vi "Add Calibration.vi"(5 "Temperature Sensors":cluster{"name":string, "reading":dbl}[](array[cluster]), 7 "Calibration Date":timestamp format="%<%x>T", 8 "error in":errorcluster, 10 "Serial Number":string, 11 "NI Skyline Configuration HTTP in":refnum<class "NI Skyline Configuration HTTP.lvclass">) -> (0 "error out":errorcluster, 3 "NI Skyline Configuration HTTP out":refnum<class "NI Skyline Configuration HTTP.lvclass">)   [LabVIEW 2020]
uses:
  <vilib>/Skyline/Configuration/Configuration HTTP_class/NI Skyline Configuration HTTP.lvclass
  <vilib>/Skyline/Configuration/Configuration HTTP_class/NI Skyline Configuration HTTP.lvclass/NI Skyline Configuration HTTP.ctl
  <vilib>/Skyline/Configuration/Configuration HTTP_class/Read Server URL.vi
  <vilib>/httpClient/POSTBuffer.vi
  <vilib>/httpClient/LabVIEWHTTPClient.lvlib
  <vilib>/addons/_JKI.lib/Serialization/JSON/JKI JSON Serialization.lvlib
panel:
  out "response headers":string
  out "response body":string
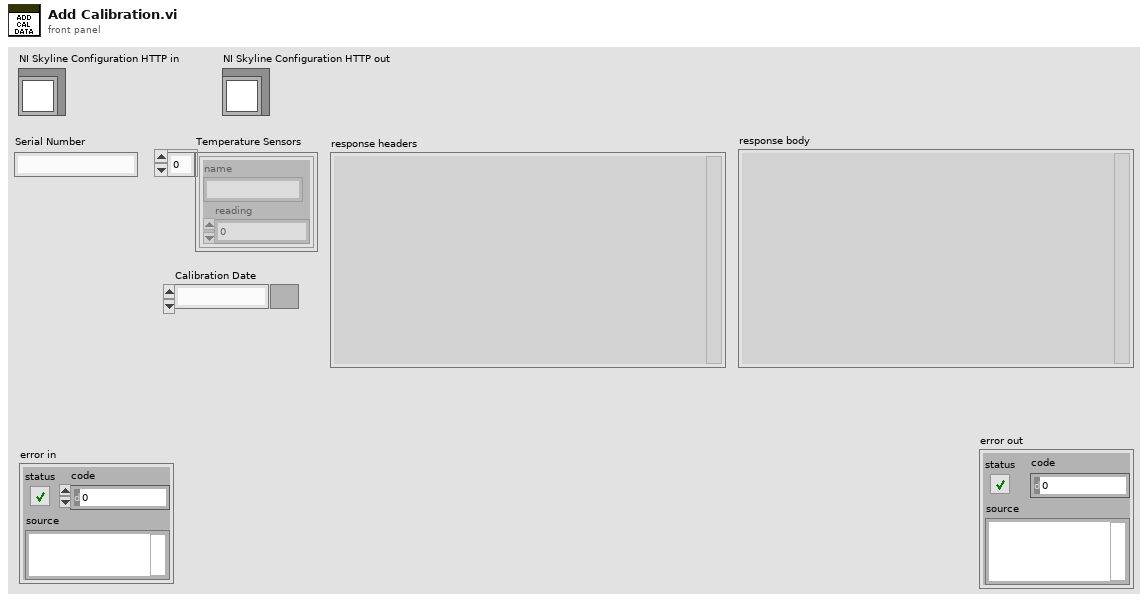
[diagram p1: front panel]
types:
  T1 = typedef "Assets.ctl" = cluster{"assets":T2[], "totalCount":u64}
  T2 = typedef "Asset.ctl" = cluster{"modelName":string, "modelNumber":u64, "serialNumber":string, "vendorName":string, "vendorNumber":u64, "busType":string, "name":string, "assetType":string, "discoveryType":string, "firmwareVersion":string, "hardwareVersion":string, "visaResourceName":string, "temperatureSensors":string[], "supportsSelfCalibration":bool, "supportsExternalCalibration":bool, "isNIAsset?":bool, "id":string, "location":cluster{"minionId":string, "parent":string, "resourceUri":string, "slotNumber":u64, "systemName":string, "state":cluster{"assetPresence":string, "systemConnection":string}}, "calibrationStatus":string, "isSystemController":bool, "externalCalibration":T3, "workspace":string, "keywords":string[], "lastUpdatedTimestamp":string}
  T3 = typedef "externalCalibration.ctl" = cluster{"temperatureSensors":cluster{"name":string, "reading":dbl}[], "isLimited":bool, "date":timestamp, "recommendedInterval":i32, "nextRecommendedDate":timestamp, "comments":string, "entrytype":string, "operator":cluster{"displayName":string, "userID":string}}
  T4 = typedef "LabVIEWHTTPClient.lvlib/ClientHandle.ctl" = refnum<k1>
  T5 = typedef "LVDateTimeRec.ctl" = cluster{"fractional second":dbl, "second":i32, "minute":i32, "hour":i32, "day of month":i32, "month":i32, "year":i32, "day of week":i32, "day of year":i32, "DST":i32}
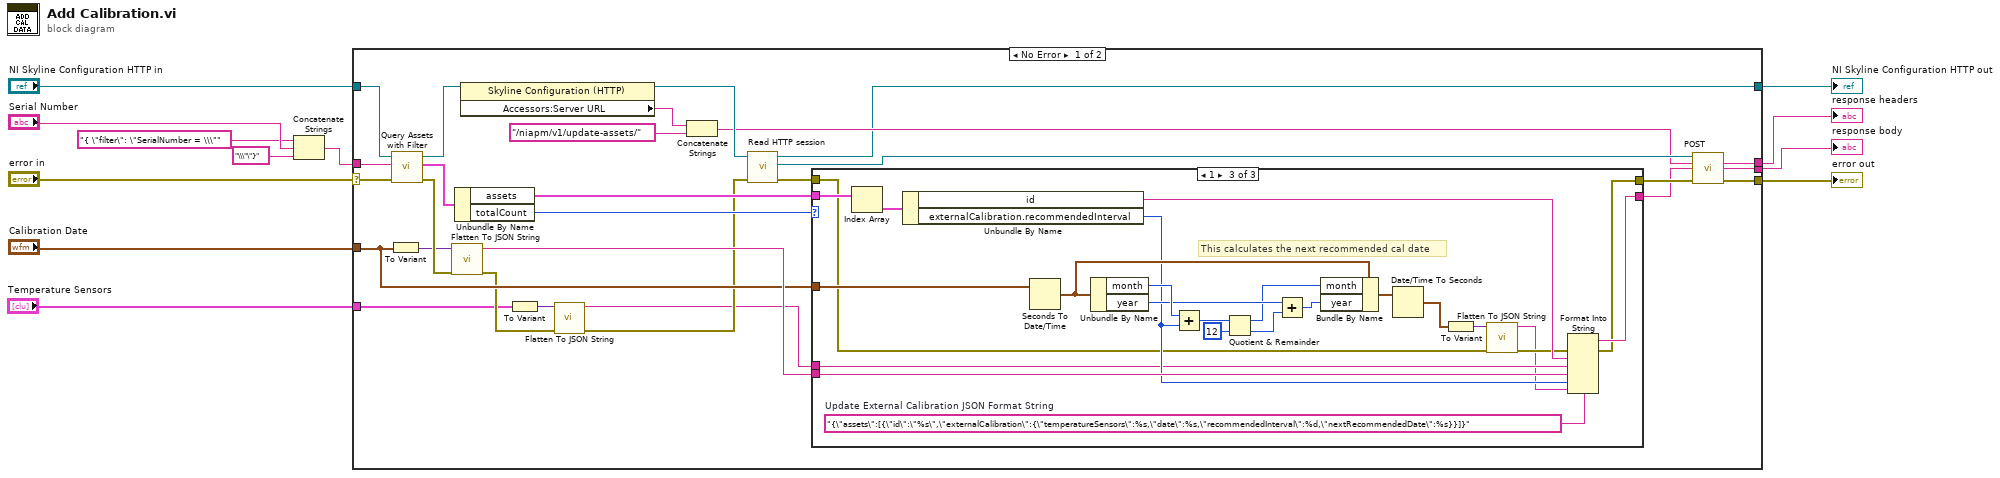
[diagram p0: block diagram]
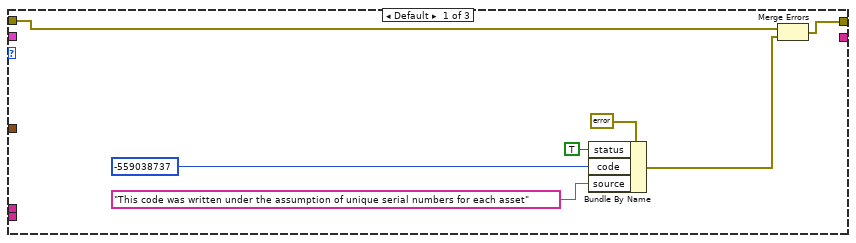
[diagram p2: hidden frame]
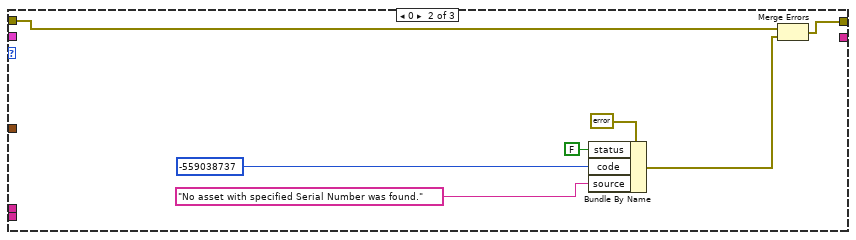
[diagram p3: hidden frame]
diagram:
  n1 = Concatenate Strings("{ \"filter\": \"SerialNumber = \\\"" ("string"), "Serial Number", "\\\"\"}" ("string")) -> (w8:string)
  n2 = case shown="No Error" "error in" {
    selector: "error in" -> [w27 w79]
    tunnel: "NI Skyline Configuration HTTP in" -> [w40 w80]
    tunnel: w8 -> [w39 _]
    tunnel: [w32 w79] -> w7
    tunnel: [w31 _] -> w6
    tunnel: [w30 w80] -> w5
    tunnel: "Calibration Date" -> [w18 _]
    tunnel: [w28 _] -> w4
    tunnel: "Temperature Sensors" -> [w14 _]
    frame No Error {
      n3 = To Variant(anything=w18) -> (Variant=w19:variant)
      n4 = call "Query Assets with Filter.vi"("Error in"=w27, "Filter string"=w39, "NI Skyline Configuration HTTP in"=w40) -> ("Error out"=w20:errorcluster, "Assets"=w29:T1, "NI Skyline Configuration HTTP out"=w38:refnum<class "NI Skyline Configuration HTTP.lvclass">)  [unwired: 6 in]
      n5 = call <vilib>:"Flatten To JSON String.vi"("error in (no error)"=w20, "Variant"=w19) -> ("error out"=w17:errorcluster, "JSON String"=w21:string)  [unwired: 8 in]
      n6 = Unbundle By Name(w29) -> ("assets"=w26:T2[], "totalCount"=w25:u64)
      n7 = property class="Skyline Configuration (HTTP)"(reference=w38) -> (reference out=w35:refnum<class "NI Skyline Configuration HTTP.lvclass">, "Accessors:Server URL"=w37:string)  [unwired: 1 in, 1 out]
      n8 = To Variant(anything=w14) -> (Variant=w15:variant)
      n9 = call <vilib>:"Flatten To JSON String.vi"("error in (no error)"=w17, "Variant"=w15) -> ("error out"=w16:errorcluster, "JSON String"=w13:string)  [unwired: 8 in]
      n10 = Concatenate Strings(w37, "/niapm/v1/update-assets/" ("initial string")) -> (w33:string)
      n11 = call <vilib>:"Read HTTP session.vi"("error in (no error)"=w16, "HTTP configuration in"=w35) -> ("error out"=w24:errorcluster, "http session"=w34:T4, "HTTP configuration out"=w30:refnum<class "NI Skyline Configuration HTTP.lvclass">)  [unwired: 7 in]
      n12 = case shown="1" w25 {
        tunnel: w26 -> [_ _ w78]
        tunnel: w18 -> [_ _ w66]
        tunnel: [_ _ w65] -> w22
        tunnel: w24 -> [w45 w52 w59]
        tunnel: [w44 w53 w64] -> w23
        tunnel: w21 -> [_ _ w63]
        tunnel: w13 -> [_ _ w61]
        frame Default {
          n13 = Bundle By Name(cluster=errorcluster {"status"=FALSE, "code"=0, "source"=""} ("error in (no error)"), "status"=TRUE, "code"=-559038737, "source"="This code was written under the assumption of unique serial numbers for each asset") -> (w47:errorcluster)
          n14 = Merge Errors(w45, w47) -> (w44:errorcluster)
        }
        frame 0 {
          n15 = Bundle By Name(cluster=errorcluster {"status"=FALSE, "code"=0, "source"=""} ("error in (no error)"), "status"=FALSE, "code"=-559038737, "source"="No asset with specified Serial Number was found.") -> (w51:errorcluster)
          n16 = Merge Errors(w52, w51) -> (w53:errorcluster)
        }
        frame 1 {
          w55 = "{\"assets\":[{\"id\":\"%s\",\"externalCalibration\":{\"temperatureSensors\":%s,\"date\":%s,\"recommendedInterval\":%d,\"nextRecommendedDate\":%s}}]}"  # Update External Calibration JSON Format String
          # "This calculates the next recommended cal date"
          n17 = Index Array(array=w78) -> (element=w77:T2)  [unwired: 1 in]
          n18 = Unbundle By Name(w77) -> ("id"=w67:string, "externalCalibration.recommendedInterval"=w62:i32)
          n19 = Seconds To Date/Time(time stamp (now)=w66) -> (date time rec=w76:T5)  [unwired: 1 in]
          n20 = Unbundle By Name(w76) -> ("month"=w75:i32, "year"=w74:i32)
          n21 = Add(x=w75, y=w62) -> (x+y=w73:i32)
          n22 = Quotient & Remainder(x=w73, y=12) -> (x-y*floor(x/y)=w70:i32, floor(x/y)=w71:i32)
          n23 = Add(x=w74, y=w71) -> (x+y=w69:i32)
          n24 = Bundle By Name(cluster=w76, "month"=w70, "year"=w69) -> (w68:T5)
          n25 = Date/Time To Seconds(2:w68) -> (0:w60:timestamp)  [unwired: 1 in]
          n26 = To Variant(anything=w60) -> (Variant=w56:variant)
          n27 = call <vilib>:"Flatten To JSON String.vi"("error in (no error)"=w59, "Variant"=w56) -> ("error out"=w58:errorcluster, "JSON String"=w57:string)  [unwired: 8 in]
          n28 = Format Into String(format string=w55, error in=w58, w67, w61, w63, w62, w57) -> (resulting string=w65:string, error out=w64:errorcluster)  [unwired: 1 in]
        }
      }
      n29 = call-poly <vilib>:"POST.vi"("client handle"=w34, "url"=w33, "buffer"=w22, "error in (no error)"=w23) -> ("headers"=w28:string, "body"=w31:string, "error out"=w32:errorcluster)  [unwired: 8 in, 1 out]
    }
    frame Error {
    }
  }
  "error out" <- w7
  "NI Skyline Configuration HTTP out" <- w5
  "response body" <- w6
  "response headers" <- w4
